vi "Get Data Channel Name.vi"(8 "error in":errorcluster, 9 "Channel Name":string, 10 "Plugin Name":string) -> (0 "error out":errorcluster, 1 "Data Channel Name":string)   [LabVIEW 2023, in "Capability.lvclass"]
uses:
  Capability.lvclass
  Capability.lvclass/Capability.ctl
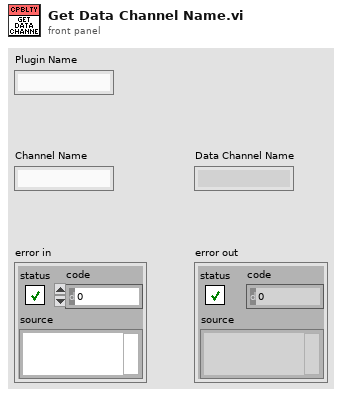
[diagram p1: front panel]
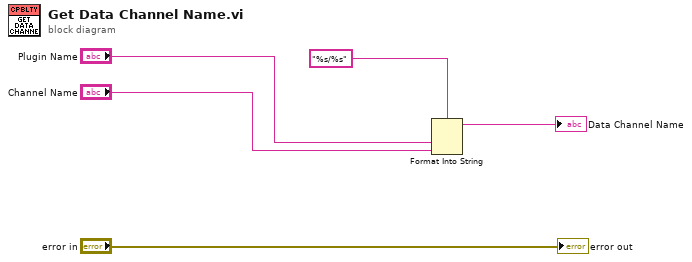
[diagram p0: block diagram]
diagram:
  n1 = Format Into String(format string="%s/%s", "Plugin Name", "Channel Name") -> (resulting string=→"Data Channel Name":string)  [unwired: 2 in, 1 out]
  "error out" <- "error in"
